vi "Averaging Previous Data.vi"() -> ()   [LabVIEW 2019]
panel:
  out "Thermometer":dbl(slide) scale=0.0..100.0
  in  "stop":bool
  # "Output\n\nLast five temperature average"
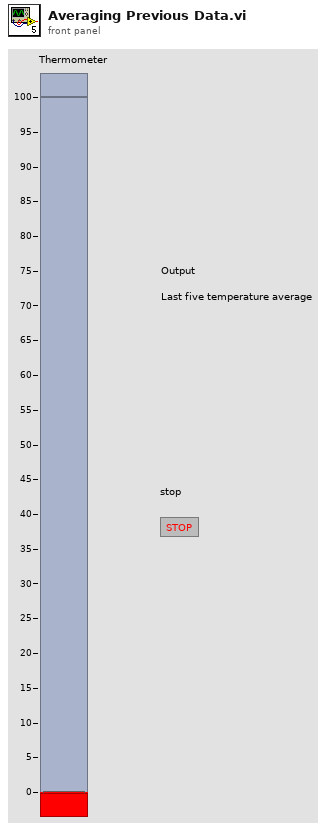
[diagram p1: front panel]
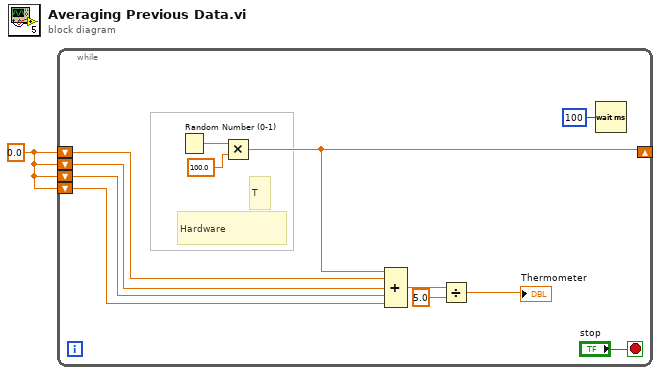
[diagram p0: block diagram]
diagram:
  w1 = 0.0
  n1 = while {
    shift-right: [w9] -> _
    shift-left: w1 -> [w8]
    shift-left: w1 -> [w7]
    shift-left: w1 -> [w6]
    shift-left: w1 -> [w5]
    stop <- "stop" stop-if-true
    # "T"
    # "Hardware"
    n2 = Random Number (0-1)() -> (number: 0 to 1=w11:dbl)
    n3 = Multiply(x=w11, y=100.0) -> (x*y=w9:dbl)
    n4 = Compound Arithmetic op=ADD(w9, w8, w7, w6, w5) -> (w4:dbl)
    n5 = Divide(x=w4, y=5.0) -> (x/y=→"Thermometer":dbl)
    n6 = Wait (ms)(milliseconds to wait=u32 100) -> ()  [unwired: 1 out]
  }
